vi "Read Inputs from system.vi"(8 "error in":errorcluster, 11 "Custom Temperature Controller runtime in":refnum<class "Custom Temperature Controller runtime.lvclass">) -> (0 "error out":errorcluster, 2 "Inputs from system":T1, 3 "Custom Temperature Controller runtime out":refnum<class "Custom Temperature Controller runtime.lvclass">)   [LabVIEW 2021, in "Custom Temperature Controller runtime.lvclass"]
uses:
  Custom Temperature Controller runtime.lvclass
  configuration/input data indices.ctl
  Custom Temperature Controller runtime.lvclass/Custom Temperature Controller runtime.ctl
  configuration/Custom Temperature Controller configuration.lvclass
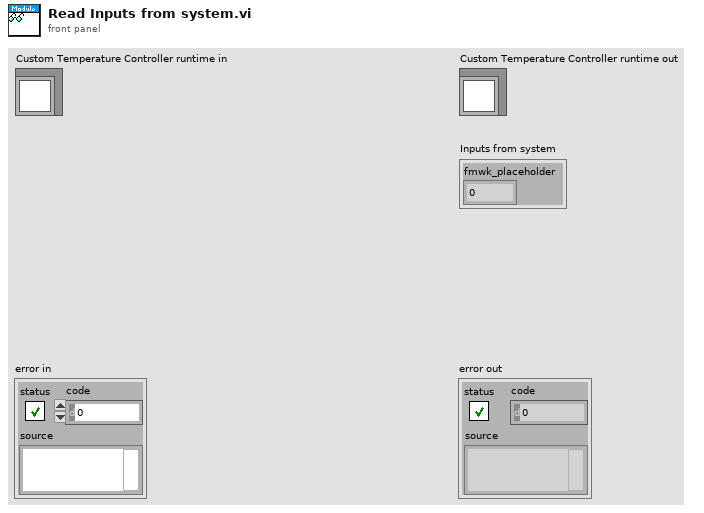
[diagram p1: front panel]
types:
  T1 = typedef "Custom Temperature Controller configuration.lvclass/input data indices.ctl" = cluster{"fmwk_placeholder":i32}
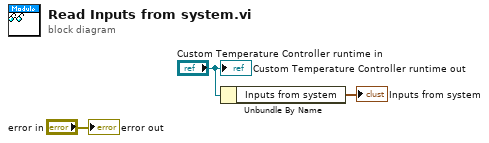
[diagram p0: block diagram]
diagram:
  n1 = Unbundle By Name("Custom Temperature Controller runtime in") -> ("Inputs from system"=→"Inputs from system":T1)
  "error out" <- "error in"
  "Custom Temperature Controller runtime out" <- "Custom Temperature Controller runtime in"
